vi "Key Down.vi"(8 "error in (no error)":errorcluster, 11 "Vk":u16) -> (0 "error out":errorcluster, 3 "INPUT":u8[](array[numeric]))   [LabVIEW 2020, in "MacroAssert.lvlib" / "Win Util.lvlib"]
uses:
  Win Util.lvlib
  Input Type.ctl
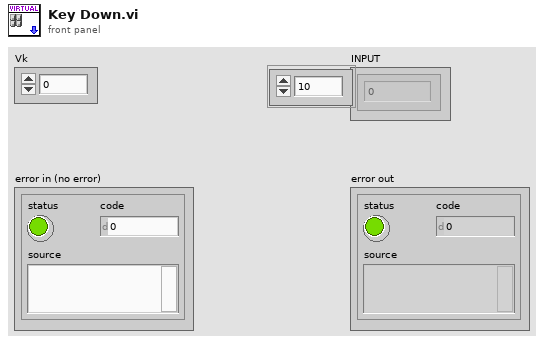
[diagram p1: front panel]
types:
  T1 = typedef "MacroAssert.lvlib/Win Util.lvlib/Input Type.ctl" = enum16{"Mouse", "Keyboard", "Hardware"}
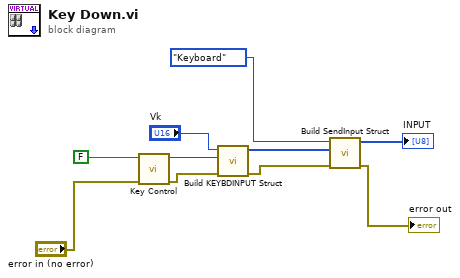
[diagram p0: block diagram]
diagram:
  n1 = call "Key Control.vi"("Error In"="error in (no error)", "KeyUp"=FALSE) -> ("Error Out"=w8:errorcluster, "Up/Down"=w1:u32)  [unwired: 8 in]
  n2 = call "Build KEYBDINPUT Struct.vi"("error in (no error)"=w8, "Flags"=w1, "Vk"="Vk") -> ("error out"=w6:errorcluster, "Array"=w4:u8[])  [unwired: 7 in]
  n3 = call "Build SendInput Struct.vi"("error in (no error)"=w6, "Data"=w4, "type"=Input_Type."Keyboard") -> ("error out"=→"error out":errorcluster, "INPUT"=→"INPUT":u8[])  [unwired: 7 in]
